vi "importExcel_DDE.vi"(1 "COLUMN":i32=1, 2 "ROW":i32=1, 3 "Filename":string="test.xls") -> (0 "Value":dbl)   [LabVIEW 2019]
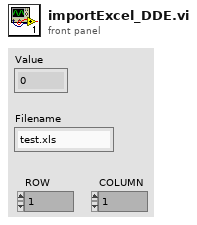
[diagram p1: front panel]
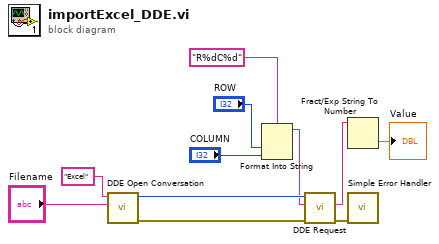
[diagram p0: block diagram]
diagram:
  n1 = call <vilib>:"DDE Open Conversation.vi"("topic"="Filename", "service"="Excel") -> ("error out"=w10:errorcluster, "conversation refnum"=w9:u32)  [unwired: 6 in]
  n2 = Format Into String(format string="R%dC%d" ("Format String"), "ROW", "COLUMN") -> (resulting string=w5:string)  [unwired: 2 in, 1 out]
  n3 = call <vilib>:"DDE Request.vi"("error in (no error)"=w10, "item"=w5, "conversation refnum in"=w9) -> ("error out"=w4:errorcluster, "data"=w3:string)  [unwired: 4 in, 1 out]
  n4 = Fract/Exp String To Number(string=w3) -> (number=→"Value":dbl)  [unwired: 3 in, 1 out]
  n5 = call <vilib>:"Simple Error Handler.vi"("error in (no error)"=w4) -> ()  [unwired: 4 in, 5 out]
